vi "Master_S.vi"() -> ()   [LabVIEW 2014]
panel:
  out "에러 출력":errorcluster
  out "숫자형 2":i32
  out "숫자형":i32
  in  "Send":bool
  out "알림 2":string
  in  "알림":string
  in  "정지":bool
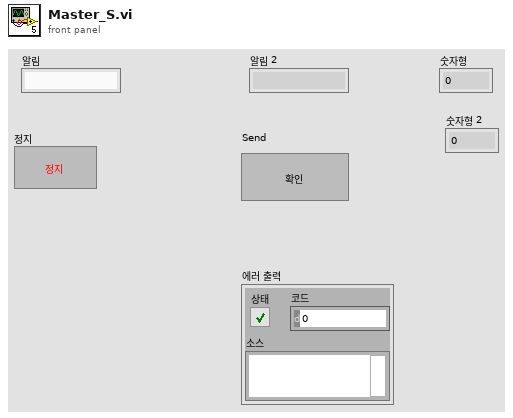
[diagram p1: front panel]
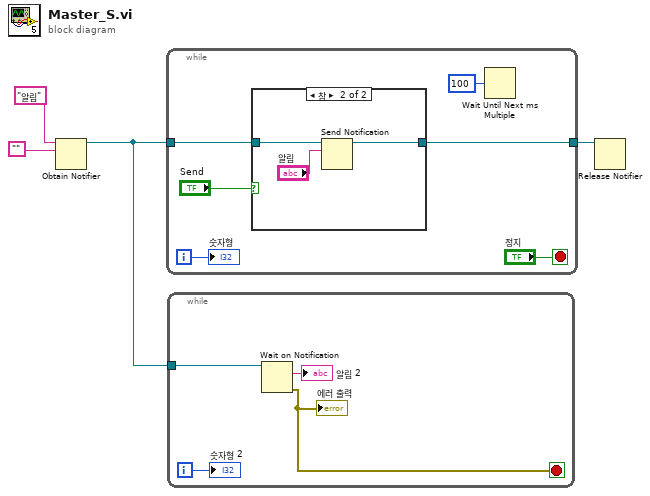
[diagram p0: block diagram]
diagram:
  n1 = Obtain Notifier(name (unnamed)="알림" ("이름(이름없음)"), notification data type="") -> (notifier out=w3:refnum<notifier>)  [unwired: 2 in, 2 out]
  n2 = while {
    tunnel: w3 -> [w8]
    tunnel: [w7] -> w4
    i -> [w5]
    stop <- "정지" stop-if-true
    n3 = case shown="참" "Send" {
      tunnel: w8 -> [w11 w14]
      tunnel: [w11 w13] -> w7
      frame False {
      }
      frame True {
        n4 = Send Notification(notification="알림", notifier=w14) -> (notifier out=w13:refnum<notifier>)  [unwired: 1 in, 1 out]
      }
    }
    n5 = Wait Until Next ms Multiple(millisecond multiple=u32 100 ("ms 배수")) -> ()  [unwired: 1 out]
    "숫자형" <- w5
  }
  n6 = while {
    tunnel: w3 -> [w18]
    i -> [w15]
    stop <- w17 stop-if-true
    n7 = Wait on Notification(notifier=w18) -> (notification=→"알림 2":string, error out=w17:errorcluster)  [unwired: 3 in, 2 out]
    "에러 출력" <- w17
    "숫자형 2" <- w15
  }
  n8 = Release Notifier(notifier=w4) -> ()  [unwired: 2 in, 3 out]
